vi "例4.3-2 比较大小（选择函数）.vi"() -> ()   [LabVIEW 2017]
panel:
  out "max":dbl
  in  "b":dbl
  in  "a":dbl
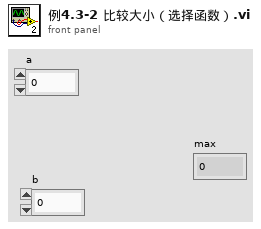
[diagram p1: front panel]
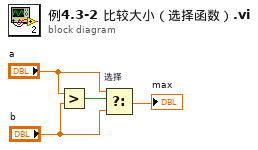
[diagram p0: block diagram]
diagram:
  n1 = Greater?(x="a", y="b") -> (0:w2:bool)
  n2 = Select "选择"(t="a", s=w2, f="b") -> (s? t:f=→"max":dbl)
